vi "習題1.vi"() -> ()   [LabVIEW 2009]
uses:
  <vilib>/NXT/Dual Mode Library/Motors/MotorCoast.vi
  <vilib>/NXT/Dual Mode Library/Waits/Wait_Rotation.vi
  <vilib>/NXT/Dual Mode Library/Motors/MotorOn.vi
  <vilib>/express/express arith-compare/Formula/XNode/ExpressFormulaBlockNode.xnode
panel:
  out "計算結果(角度)":dbl
  in  "輪胎半徑":dbl
  in  "行進距離(cm)":dbl
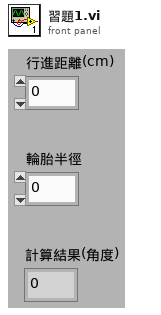
[diagram p1: front panel]
types:
  T1 = typedef "LVHSConnector.ctl" = cluster{"error":errorcluster, "address":string, "NXT #":i32, "Show Error":bool, "Connection":u16}
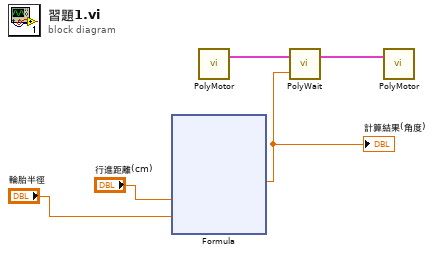
[diagram p0: block diagram]
diagram:
  n1 = xnode "Formula"("X"="行進距離(cm)", "Y"="輪胎半徑") -> ("Result"=w3:dbl)  [unwired: 1 in, 1 out]
  "計算結果(角度)" <- w3
  n2 = call-poly <vilib>:"PolyMotor.vi"() -> ("NXT"=w4:T1)  [unwired: 4 in]
  n3 = call-poly <vilib>:"PolyWait.vi"("Position Change (180)"=w3, "NXT"=w4) -> ("NXT"=w5:T1)  [unwired: 2 in]
  n4 = call-poly <vilib>:"PolyMotor.vi"("NXT"=w5) -> ()  [unwired: 3 in, 1 out]
